vi "Valve Control Single 6008.vi"(8 "error in":errorcluster, 9 "Valve On?":bool, 10 "Valve Number":i32, 11 "Port":tag="Dev2/port0") -> (0 "error out":errorcluster)   [LabVIEW 2012]
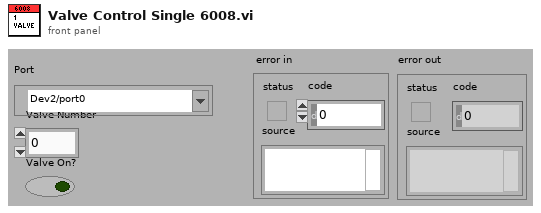
[diagram p1: front panel]
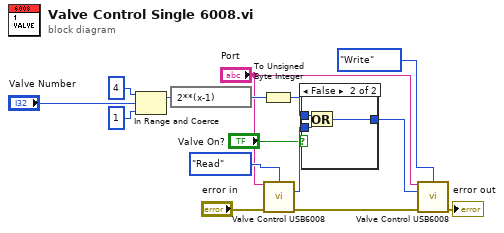
[diagram p0: block diagram]
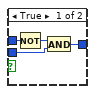
[diagram p2: hidden frame]
diagram:
  n1 = In Range and Coerce(upper limit=4, x="Valve Number", lower limit=1) -> (coerced(x)=w10:i32)  [unwired: 1 out]
  n2 = expression code="2**(x-1)"(w10) -> (w9:i32)
  n3 = To Unsigned Byte Integer(number=w9) -> (unsigned 8bit integer=w7:u8)
  n4 = call "Valve Control USB6008.vi"("Port"="Port", "Mode"=enum16{"Read", "Write"}."Read", "error in"="error in") -> ("Data"=w14:u8, "error out"=w2:errorcluster)  [unwired: 11 in]
  n5 = case shown="False" "Valve On?" {
    tunnel: w14 -> [w19 w22]
    tunnel: [w18 w21] -> w8
    tunnel: w7 -> [w17 w20]
    frame True {
      n6 = Not(x=w17) -> (.not. x?=w16:u8)
      n7 = And(x=w16, y=w19) -> (x .and. y?=w18:u8)
    }
    frame False {
      n8 = Or(x=w20, y=w22) -> (x .or. y?=w21:u8)
    }
  }
  n9 = call "Valve Control USB6008.vi"("Port"="Port", "Mode"=enum16{"Read", "Write"}."Write", "Write Val"=w8, "error in"=w2) -> ("error out"=→"error out":errorcluster)  [unwired: 10 in, 1 out]
